vi "Configure Aperture.vi"(7 "Auto Aperture (0: OFF)":i32(ring) items=["OFF", "ON", "ONCE"], 8 "error in (no error)":errorcluster, 9 "Aperture Integration Time (1.6667000000E-2 s)":dbl=0.016667 format="%.10e", 10 "Measurement Function (0: Voltage)":i32(ring) items=["Voltage", "Current", "Resistance", "Charge"], 11 "VISA resource name":refnum<visa-resource-name>) -> (0 "error out":errorcluster, 3 "VISA resource name out":refnum<visa-resource-name>)   [LabVIEW 2016, in "Keithley 6517.lvlib"]
doc: "Configures the aperture settings for the measurement functions (Voltage, Current, Resistance and Charge).\n\nNote:\nThe specified measurement should be enabled from <b>Configure Measurement Function.vi</b>.\n\nThis VI is <B>NOT</B> compatible with model <B>6514</B>."
uses:
  <instrlib>/Keithley 6517/Keithley 6517.lvlib
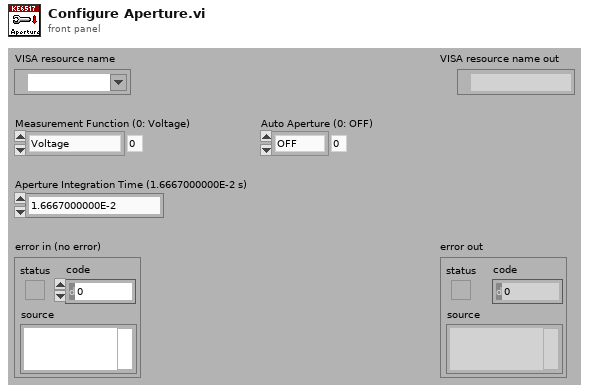
[diagram p1: front panel]
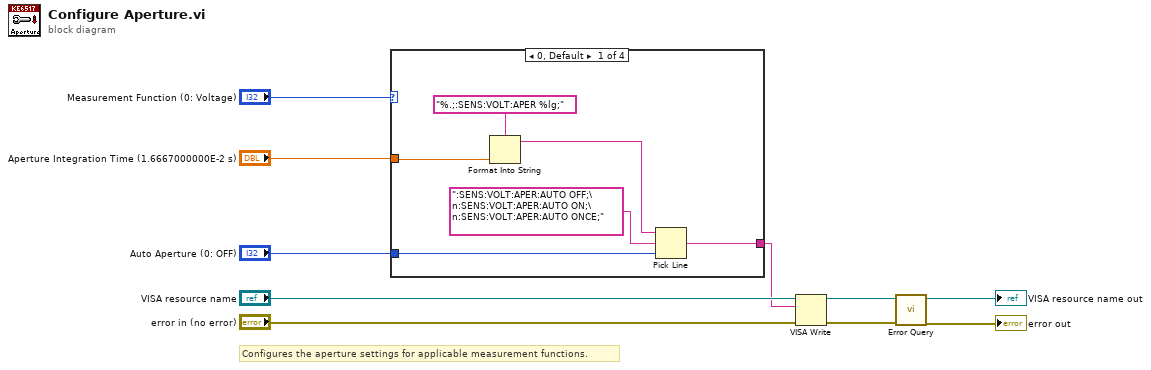
[diagram p0: block diagram]
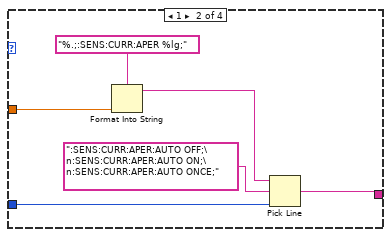
[diagram p2: hidden frame]
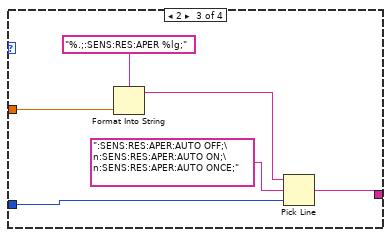
[diagram p3: hidden frame]
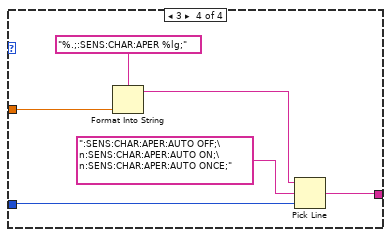
[diagram p4: hidden frame]
diagram:
  # "Configures the aperture settings for applicable measurement functions."
  n1 = case shown="0, Default" "Measurement Function (0: Voltage)" {
    tunnel: "Aperture Integration Time (1.6667000000E-2 s)" -> [w15 w21 w27 w33]
    tunnel: "Auto Aperture (0: OFF)" -> [w14 w20 w25 w31]
    tunnel: [w12 w18 w26 w32] -> w2
    frame 0, Default {
      n2 = Format Into String(format string="%.;:SENS:VOLT:APER %lg;", w15) -> (resulting string=w11:string)  [unwired: 2 in, 1 out]
      n3 = Pick Line(string ("")=w11, multi-line string=":SENS:VOLT:APER:AUTO OFF;\n:SENS:VOLT:APER:AUTO ON;\n:SENS:VOLT:APER:AUTO ONCE;", line index=w14) -> (output string=w12:string)
    }
    frame 1 {
      n4 = Format Into String(format string="%.;:SENS:CURR:APER %lg;", w21) -> (resulting string=w17:string)  [unwired: 2 in, 1 out]
      n5 = Pick Line(string ("")=w17, multi-line string=":SENS:CURR:APER:AUTO OFF;\n:SENS:CURR:APER:AUTO ON;\n:SENS:CURR:APER:AUTO ONCE;", line index=w20) -> (output string=w18:string)
    }
    frame 2 {
      n6 = Format Into String(format string="%.;:SENS:RES:APER %lg;", w27) -> (resulting string=w23:string)  [unwired: 2 in, 1 out]
      n7 = Pick Line(string ("")=w23, multi-line string=":SENS:RES:APER:AUTO OFF;\n:SENS:RES:APER:AUTO ON;\n:SENS:RES:APER:AUTO ONCE;", line index=w25) -> (output string=w26:string)
    }
    frame 3 {
      n8 = Format Into String(format string="%.;:SENS:CHAR:APER %lg;", w33) -> (resulting string=w29:string)  [unwired: 2 in, 1 out]
      n9 = Pick Line(string ("")=w29, multi-line string=":SENS:CHAR:APER:AUTO OFF;\n:SENS:CHAR:APER:AUTO ON;\n:SENS:CHAR:APER:AUTO ONCE;", line index=w31) -> (output string=w32:string)
    }
  }
  n10 = VISA Write(VISA resource name="VISA resource name", write buffer=w2, error in (no error)="error in (no error)") -> (VISA resource name out=w9:refnum<visa-resource-name>, error out=w8:errorcluster)  [unwired: 1 out]
  n11 = call <instrlib>:"Error Query.vi"("error in (no error)"=w8, "VISA resource name"=w9) -> ("error out"=→"error out":errorcluster, "VISA resource name out"=→"VISA resource name out":refnum<visa-resource-name>)  [unwired: 6 in, 2 out]
